vi "RSZVB Edit Limit Line Segment.vi"(0 "VISA session":refnum<visa-resource-name>, 1 "Stop Stimulus (0.0)":dbl format="%^.3e", 2 "Stop Response (0.0)":dbl format="%^.3e", 5 "Channel (Trace) (1)":i32=1, 7 "Segment (1)":i32=1, 9 "Type (1: Upper)":i32(ring)=1 items=["Off", "Upper", "Lower"], 11 "error in (no error)":errorcluster {"code" format="%.0x"}, 12 "Start Response (0.0)":dbl format="%^.3e", 13 "Start Stimulus (0.0)":dbl format="%^.3e") -> (4 "dup VISA session":refnum<visa-resource-name>, 15 "error out":errorcluster {"code" format="%.0x"})   [LabVIEW 2011]
doc: "This VI edits existing segment of the limit line segments list.\n\nNote(s):\n\nA segment must be created first to enable this VI.\n\nRemote-control command(s):\nCALCulate<Ch/Tr>:LIMit:SEGMent<Seg>:TYPE LMIN | LMAX | OFF\nCALCulate<Ch/Tr>:LIMit:SEGMent<Seg>:STIMulus:STARt <numeric_value>\nCALCulate<Ch/Tr>:LIMit:SEGMent<Seg>:STIMulus:STOP <numeric_value>\nCALCulate<Ch/Tr>:LIMit:SEGMent<Seg>:AMPLitude:STARt <numeric_value>\nCALCulate<Ch/Tr>:LIMit:SEGMent<Seg>:AMPLitude:STOP <numeric_value>"
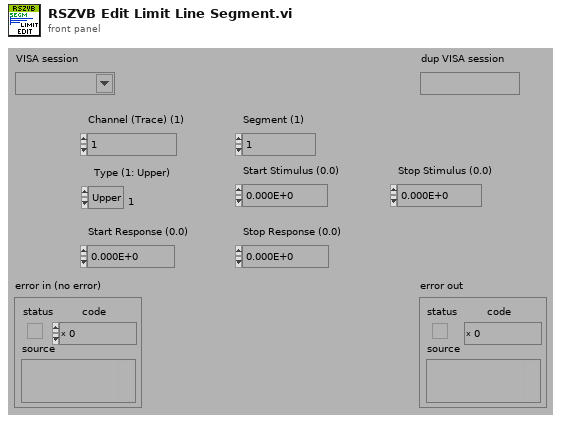
[diagram p1: front panel]
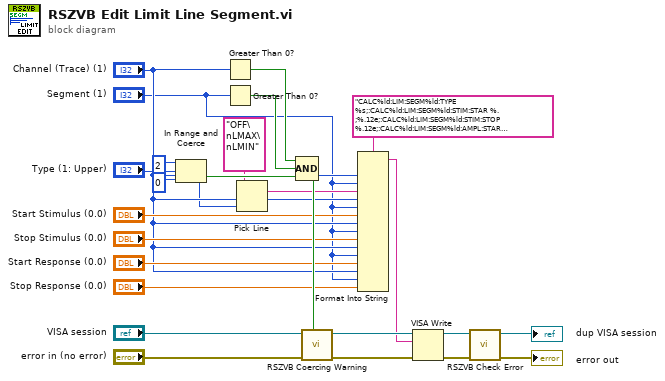
[diagram p0: block diagram]
diagram:
  n1 = In Range and Coerce(upper limit=2, x="Type (1: Upper)", lower limit=0) -> (coerced(x)=w2:i32, In Range?=w19:bool)
  n2 = Greater Than 0?(x="Channel (Trace) (1)") -> (x > 0?=w15:bool)
  n3 = Greater Than 0?(x="Segment (1)") -> (x > 0?=w14:bool)
  n4 = Pick Line(multi-line string="OFF\nLMAX\nLMIN", line index=w2) -> (output string=w13:string)  [unwired: 1 in]
  n5 = Compound Arithmetic op=AND(w15, w14, w19) -> (w18:bool)
  n6 = call "RSZVB Coercing Warning.vi"("In Range?"=w18, "error in (no error)"="error in (no error)", "VISA session"="VISA session") -> ("error out"=w25:errorcluster, "dup VISA session"=w26:refnum<visa-resource-name>)  [unwired: 7 in]
  n7 = Format Into String(format string="CALC%ld:LIM:SEGM%ld:TYPE %s;:CALC%ld:LIM:SEGM%ld:STIM:STAR %.;%.12e;:CALC%ld:LIM:SEGM%ld:STIM:STOP %.12e;:CALC%ld:LIM:SEGM%ld:AMPL:STAR %.12e;:CALC%ld:LIM:SEGM%ld:AMPL:STOP %.12e", "Channel (Trace) (1)", "Segment (1)", w13, "Channel (Trace) (1)", "Segment (1)", "Start Stimulus (0.0)", "Channel (Trace) (1)", "Segment (1)", "Stop Stimulus (0.0)", "Channel (Trace) (1)", "Segment (1)", "Start Response (0.0)", "Channel (Trace) (1)", "Segment (1)", "Stop Response (0.0)") -> (resulting string=w17:string)  [unwired: 2 in, 1 out]
  n8 = VISA Write(VISA resource name=w26, write buffer=w17, error in (no error)=w25) -> (VISA resource name out=w23:refnum<visa-resource-name>, error out=w24:errorcluster)  [unwired: 1 out]
  n9 = call "RSZVB Check Error.vi"("error in (no error)"=w24, "VISA session"=w23) -> ("error out"=→"error out":errorcluster, "dup VISA session"=→"dup VISA session":refnum<visa-resource-name>)  [unwired: 8 in]
